vi "main.vi"() -> ()   [LabVIEW 2018]
uses:
  typedefs/measurement_settings.ctl
  typedefs/device_details.ctl
  typedefs/state_selector.ctl
  <instrlib>/Keithley 24XX/Public/Data/Read (Multiple Points).vi
  <instrlib>/Keithley 24XX/Keithley 24XX.lvlib
panel:
  out "timestamp":string
  out "experiment folder":path
  out "settings path":path
  out "Pixel data file":path
  in  "Tab Control":enum32{"Settings", "Measurement", "Advanced"}(tab)
  in  "Device details":T1={"Device label"="", "Pixel"=enum."1", "Area (cm^2)"=0.0}
  out "Username":string
  out "Experiment Name":string
  in  "Measurement settings":T2={"Minimum LED current (A)"=0.001, "Maximum LED Current (A)"=0.7, "Number of LED currents in sweep"=20, "LED current sweep mode"=1, "LED current sweep direction"=0, "LED settling delay (ms)"=500, "Solar cell measurement mode"=0, "Minimum JV voltage (V)"=-1.2, "Maximum JV voltage (V)"=0.1, "JV voltage step (V)"=0.02, "JV sweep direction"=0, "Dual JV sweep"=1, "Current range"=0, "Voltage range"=2, "Integration time (NPLC)"=1, "Auto settling delay"=1, "Settling delay (ms)"=3.0, "Enable display"=0} {"Voltage range" items=["Auto", "200 mV", "2.1 V", "21 V", "210 V"]; "Enable display" items=["False", "True"]; "Auto settling delay" items=["False", "True"]; "Settling delay (ms)" min=0.2 max=999999.9; "Integration time (NPLC)" items=["0.01", "0.1", "1", "10"]; "Current range" items=["Auto", "1 uA", "10 uA", "100 uA", "1 mA", "10 mA", "100 mA", "1 A"]; "Dual JV sweep" items=["False", "True"]; "JV sweep direction" items=["Ascending", "Descending"]; "JV voltage step (V)" min=0.0001 max=5.0 step=0.0001; "Solar cell measurement mode" items=["J-V", "Voc", "Jsc"]; "LED current sweep direction" items=["Ascending", "Descending"]; "LED current sweep mode" items=["Linear", "Logarithmic"]; "Maximum LED Current (A)" min=0.0 max=0.7 step=0.001 format="%#.3f"; "Minimum LED current (A)" min=0.0 max=0.7 step=0.001 format="%#.3f"}
  in  "Scan":bool
  in  "Initialise instruments":bool
  in  "Stop scan":bool
  out "TTi Power Supply":bool
  out "Pixel Selector":bool
  in  "Exit":bool
  out "Kiethley 2400":bool
  in  "LED current (A)":dbl=0.1 min=0.0 max=0.5
  in  "Pixel":u16=1
  out "Light on":bool
  in  "Toggle white light":bool
  in  "Keithley Address":refnum<visa-resource-name>="GPIB0::8::INSTR"
  in  "TTi QL564P":refnum<visa-resource-name>="COM6"
  in  "Set switch":bool
  in  "Tab Control 2":enum32{"Page 1"}(tab)
  out "Graph":cluster{"Voltage":dbl[], dbl[]}[](graph)
  # "Intensity Dependence"
  # "1."
  # "4."
  # "5."
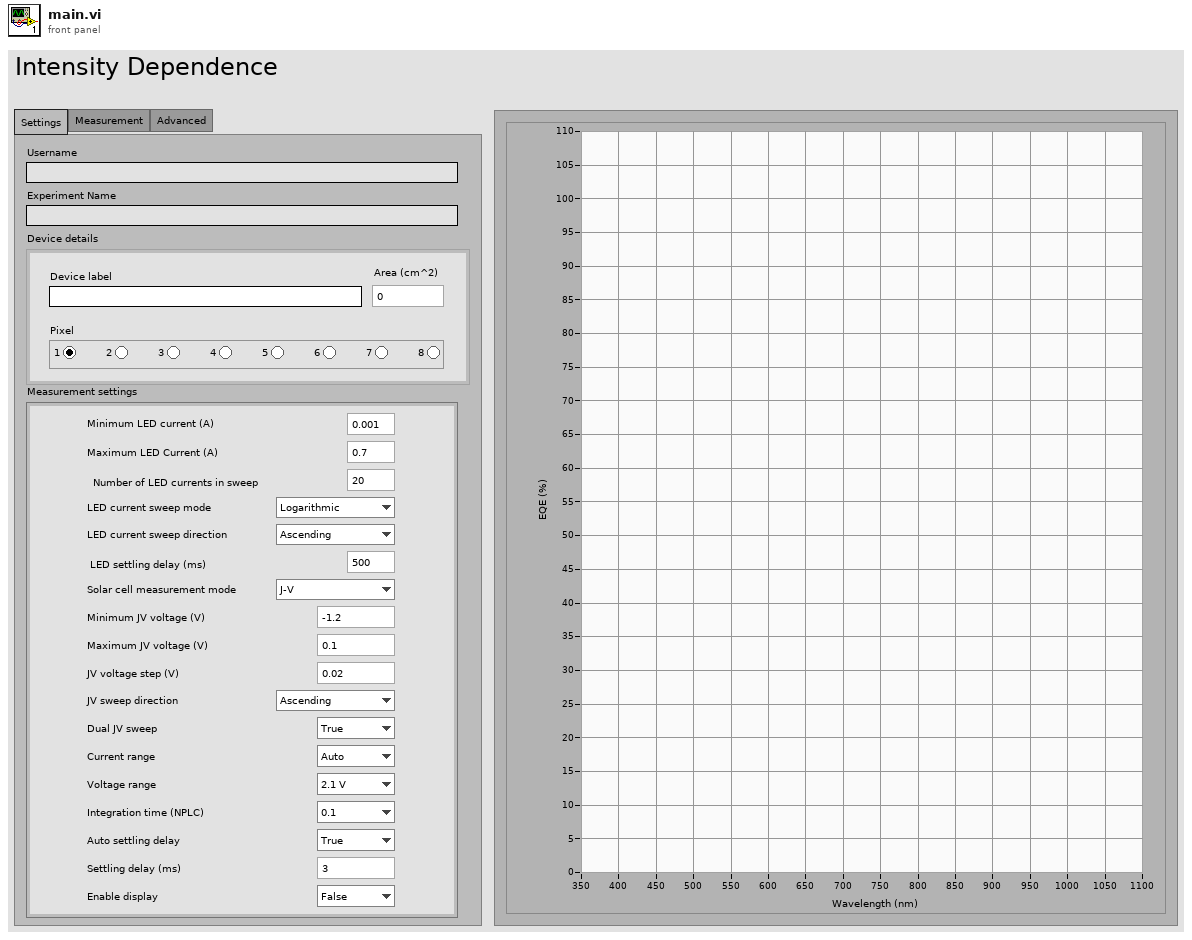
[diagram p1: front panel]
types:
  T1 = typedef "device_details.ctl" = cluster{"Device label":string, "Pixel":enum32{"No Selection", "1", "2", "3", "4", "5", "6", "7", "8"}, "Area (cm^2)":dbl}
  T2 = typedef "measurement_settings.ctl" = cluster{"Minimum LED current (A)":dbl, "Maximum LED Current (A)":dbl, "Number of LED currents in sweep":u32, "LED current sweep mode":u16, "LED current sweep direction":u16, "LED settling delay (ms)":u32, "Solar cell measurement mode":u16, "Minimum JV voltage (V)":dbl, "Maximum JV voltage (V)":dbl, "JV voltage step (V)":dbl, "JV sweep direction":u16, "Dual JV sweep":u16, "Current range":u16, "Voltage range":u16, "Integration time (NPLC)":u16, "Auto settling delay":u16, "Settling delay (ms)":dbl, "Enable display":u16}
  T3 = typedef "state_selector.ctl" = enum16{"Initialise software", "Idle", "Initialise instruments", "Scan", "Exit"}
  T4 = enum8{"Enabled", "Disabled", "Disabled and Grayed Out"}
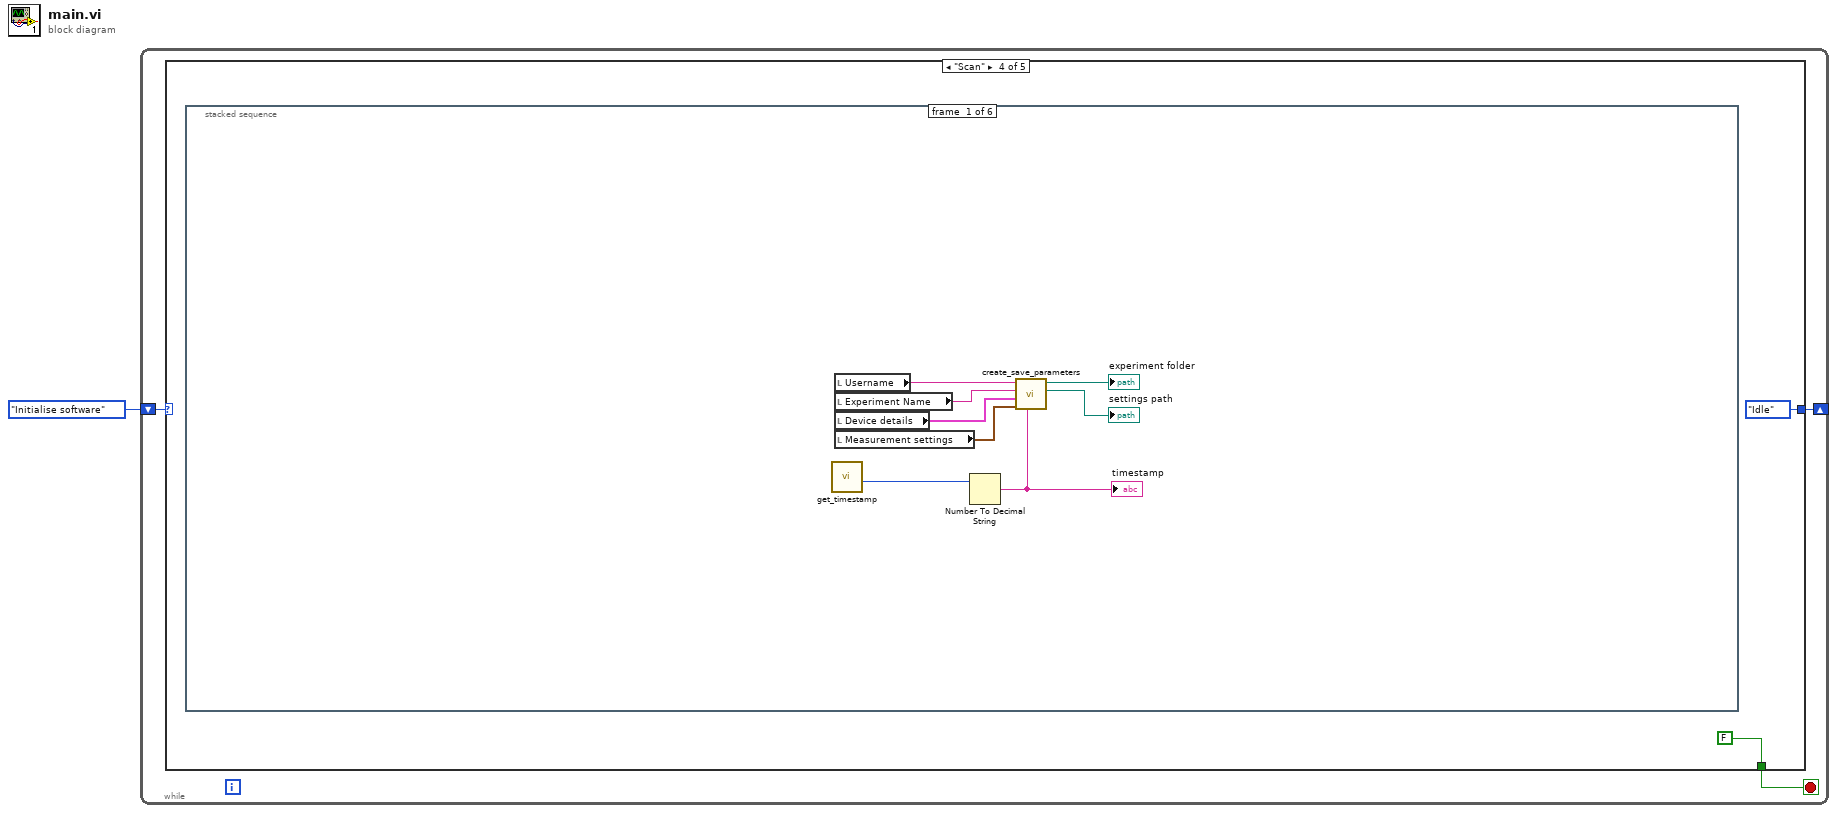
[diagram p0: block diagram]
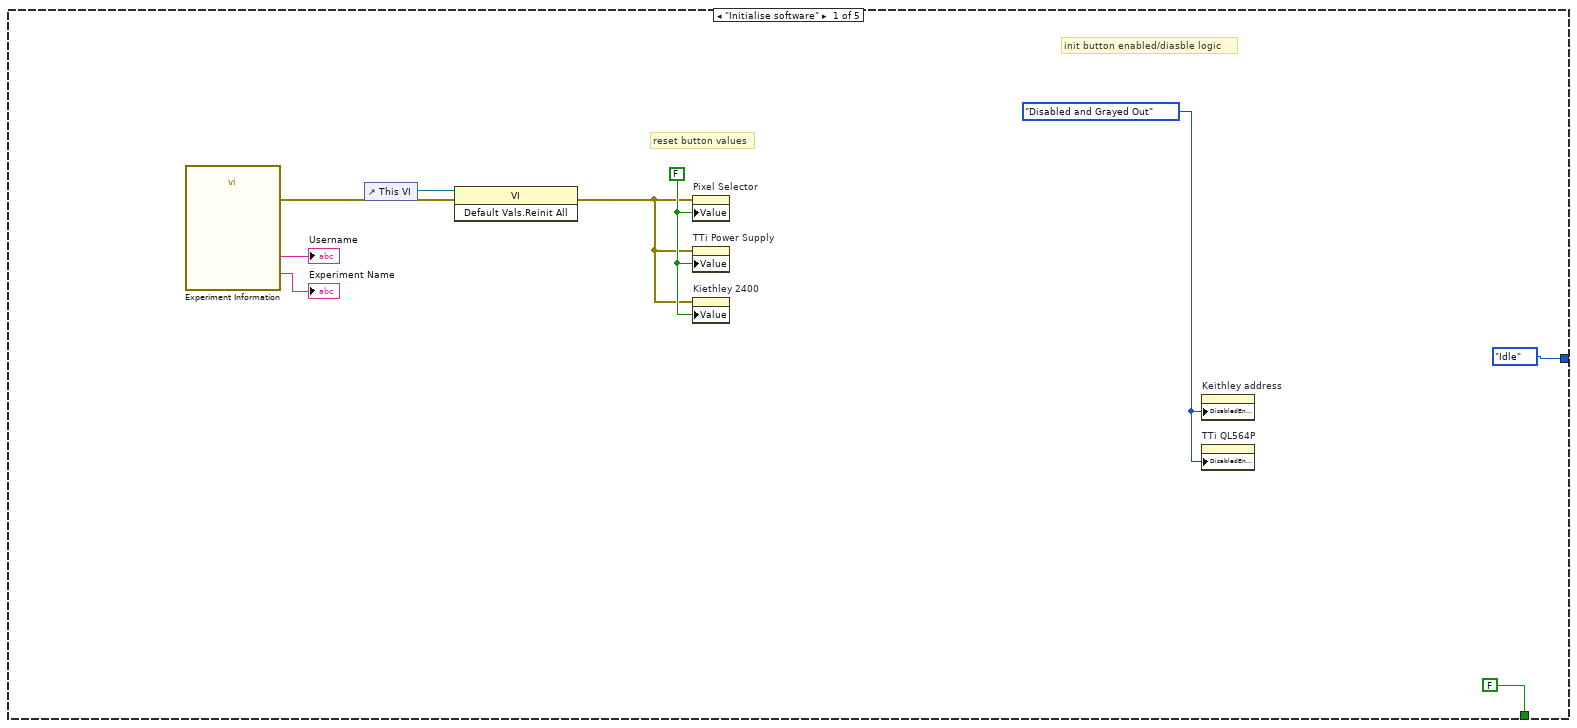
[diagram p2: hidden frame]
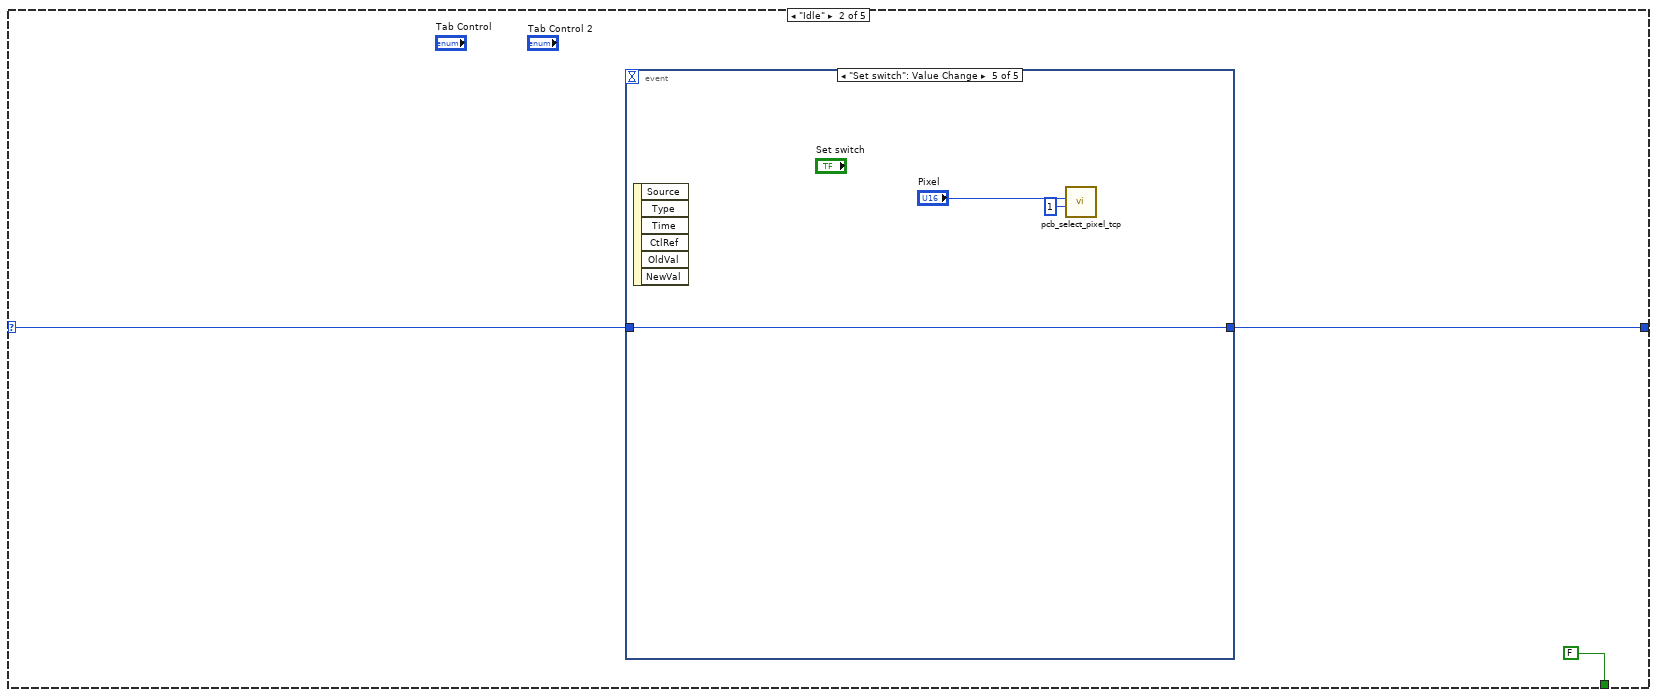
[diagram p3: hidden frame]
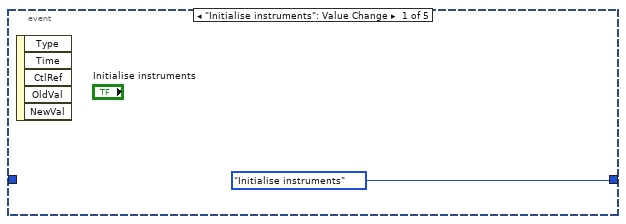
[diagram p4: hidden frame]
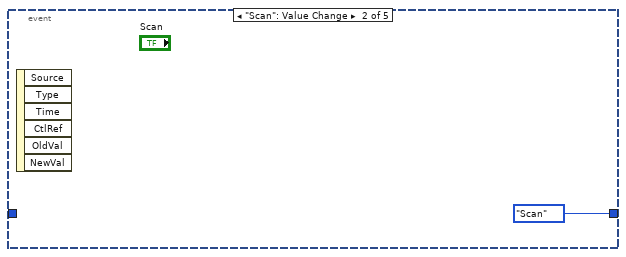
[diagram p5: hidden frame]
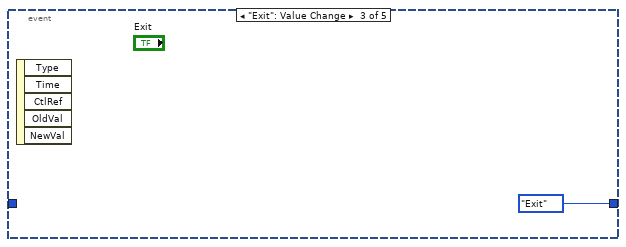
[diagram p6: hidden frame]
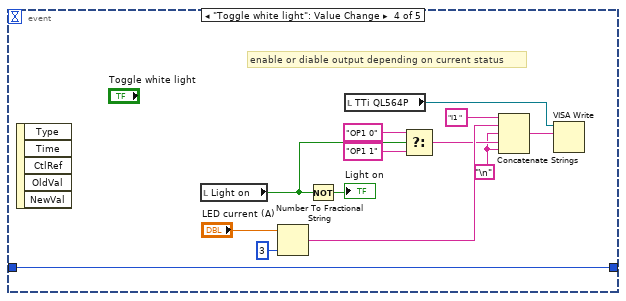
[diagram p7: hidden frame]
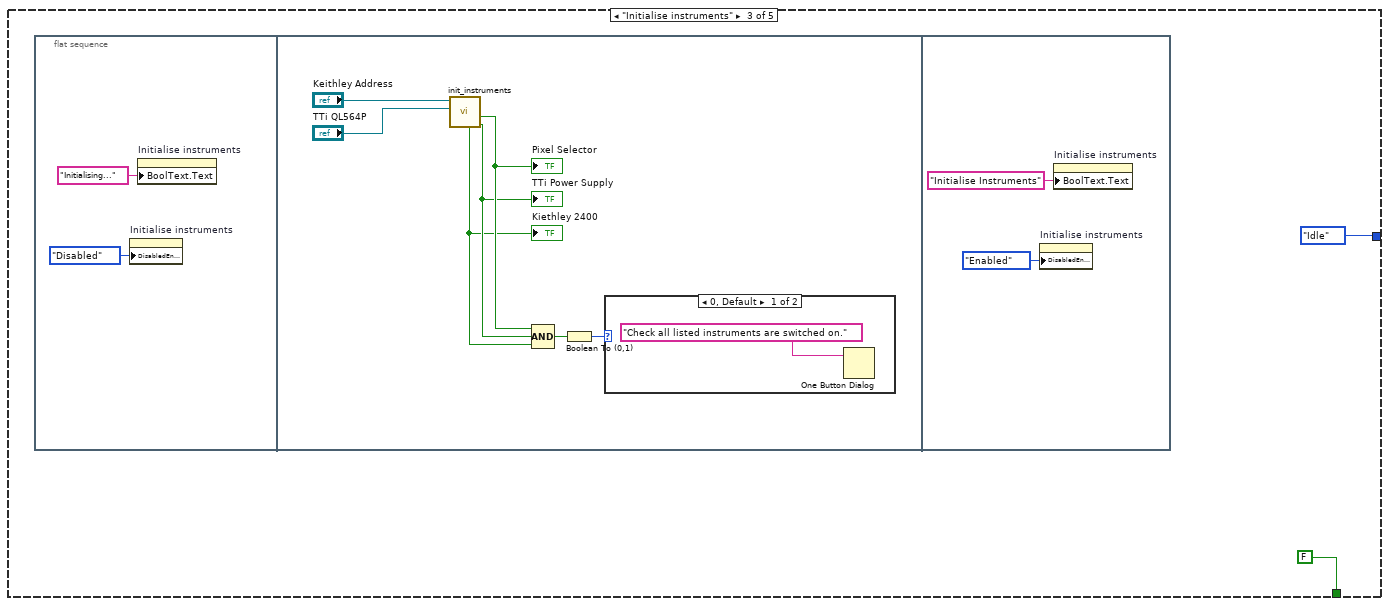
[diagram p8: hidden frame]
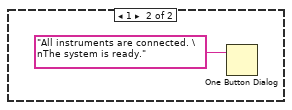
[diagram p9: hidden frame]
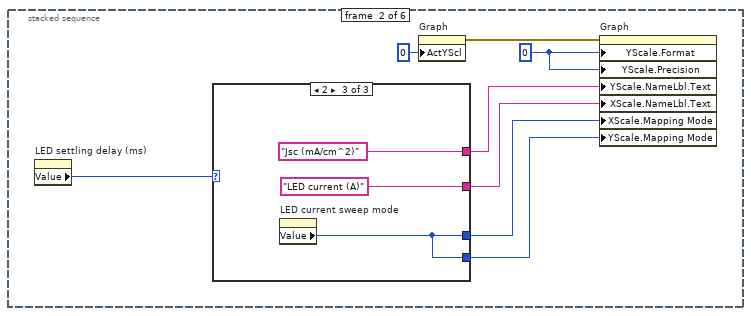
[diagram p10: hidden frame]
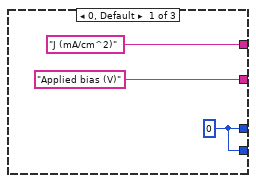
[diagram p11: hidden frame]
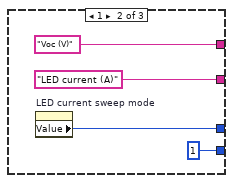
[diagram p12: hidden frame]
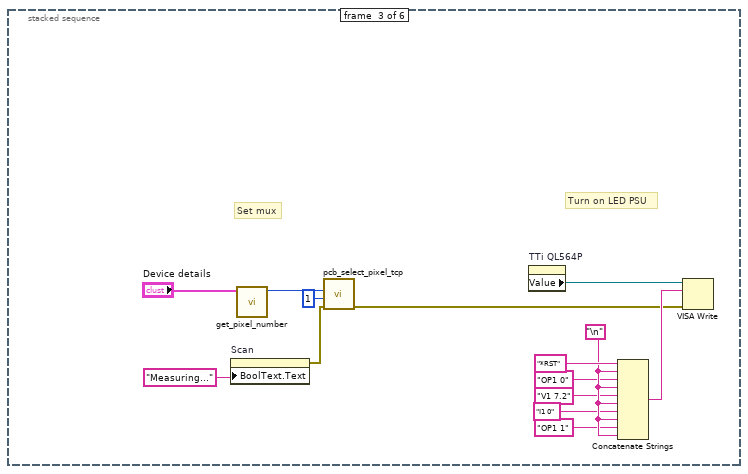
[diagram p13: hidden frame]
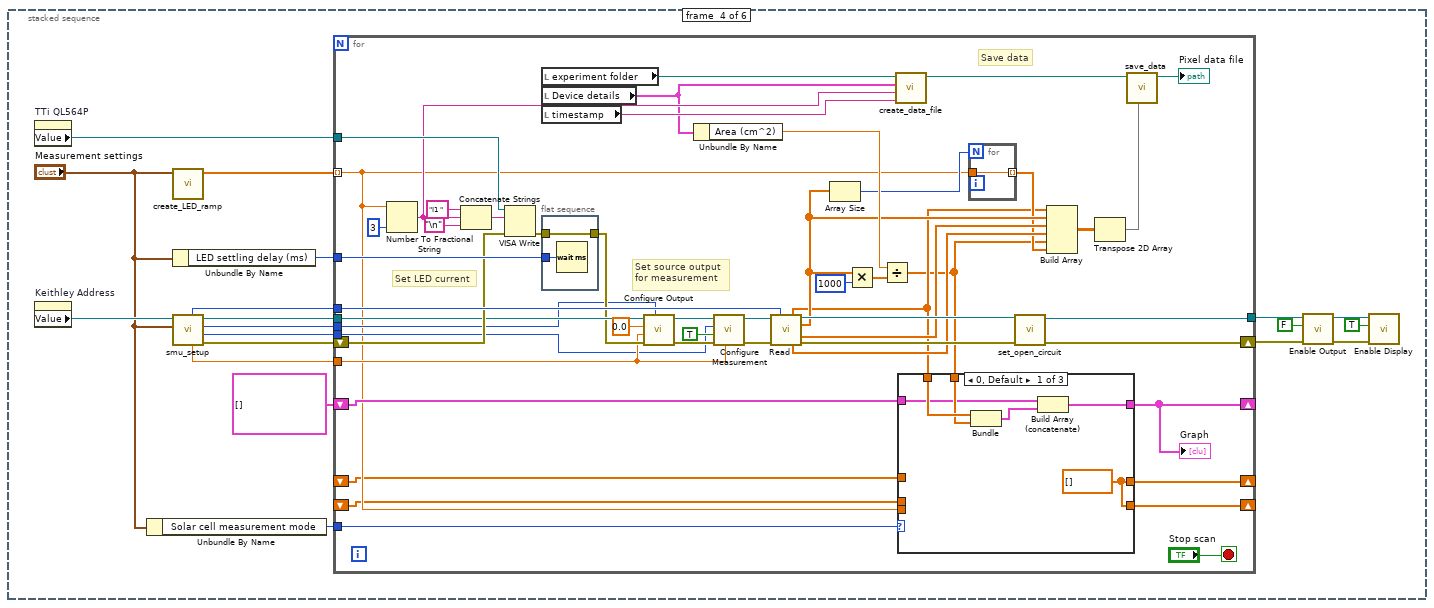
[diagram p14: hidden frame]
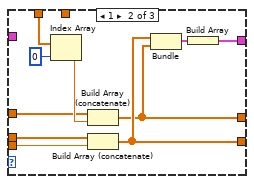
[diagram p15: hidden frame]
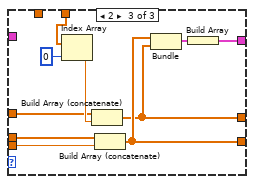
[diagram p16: hidden frame]
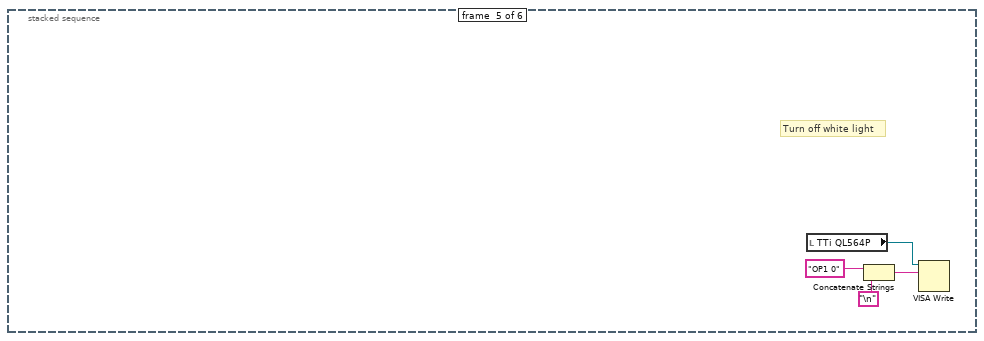
[diagram p17: hidden frame]
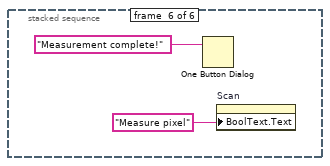
[diagram p18: hidden frame]
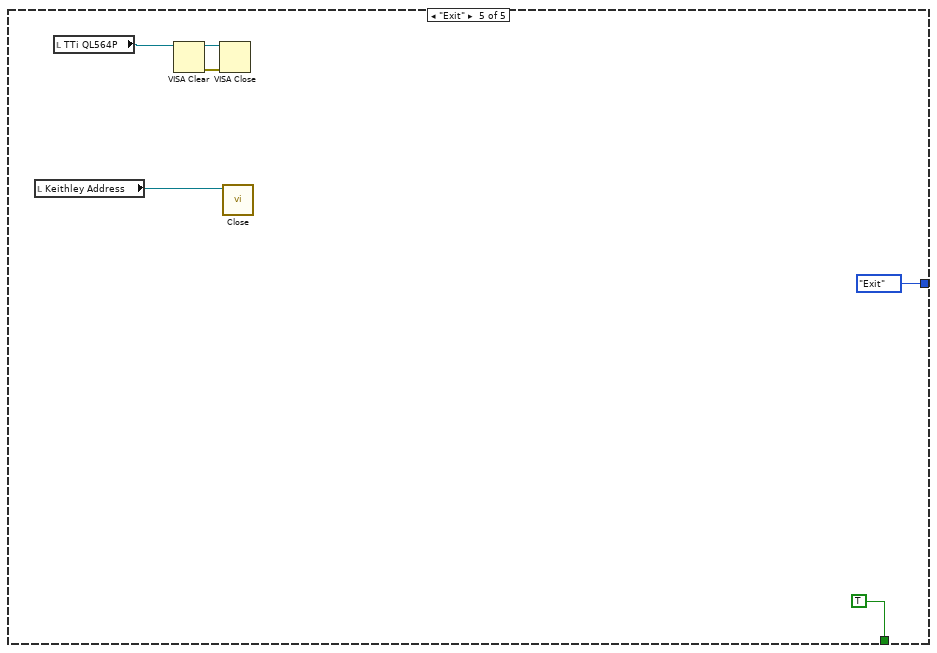
[diagram p19: hidden frame]
diagram:
  n1 = while {
    shift-right: [w3] -> _
    shift-left: state_selector."Initialise software" ("Enum") -> [w4]
    stop <- w2 stop-if-true
    n2 = case shown="\"Scan\"" w4 {
      selector: w4 -> [_ w15 _ _ _]
      tunnel: [state_selector."Idle" ("Enum") w16 state_selector."Idle" ("Enum") state_selector."Idle" ("Enum") state_selector."Exit" ("Enum")] -> w3
      tunnel: [FALSE FALSE FALSE FALSE TRUE] -> w2
      frame "Initialise software" {
        w8 = T4."Disabled and Grayed Out" ("Disabled")
        w9 = FALSE ("Scan")
        # "init button enabled/diasble logic"
        # "reset button values"
        n3 = call "Experiment Information"() -> ("Experiment Title"=→"Experiment Name":string, "Username"=→"Username":string, "error out"=w6:errorcluster)  [unwired: 16 in, 1 out]
        n4 = control-ref of="This VI"() -> (w7:refnum<vi>)
        n5 = invoke class="VI" method="Default Vals.Reinit All"(reference=w7, error in=w6) -> (error out=w5:errorcluster)  [unwired: 1 in, 2 out]
        n6 = property on="Pixel Selector" class="Bool (strict)"(error in=w5, "Value"=w9) -> ()  [unwired: 1 in, 2 out]
        n7 = property on="TTi Power Supply" class="Bool (strict)"(error in=w5, "Value"=w9) -> ()  [unwired: 1 in, 2 out]
        n8 = property on="Kiethley 2400" class="Bool (strict)"(error in=w5, "Value"=w9) -> ()  [unwired: 1 in, 2 out]
        n9 = property on="Keithley address" class="VISAName"("DisabledEnum"=w8) -> ()  [unwired: 2 in, 2 out]
        n10 = property on="TTi QL564P" class="VISAName"("DisabledEnum"=w8) -> ()  [unwired: 2 in, 2 out]
      }
      frame "Idle" {
        n11 = event shown="[4] \"Set switch\": Value Change" {
          selector: _ -> [_ _ _ _ _]
          dyn-events: _ -> [_ _ _ _ _]
          timeout: _ -> [_ _ _ _ _]
          tunnel: w15 -> [_ _ _ w32 w35]
          tunnel: [state_selector."Initialise instruments" ("Enum") state_selector."Scan" ("Enum") state_selector."Exit" ("Enum") w32 w35] -> w16
          event "Initialise instruments": Value Change {
            n12 = event-data() -> ()  [unwired: 1 in, 5 out]
          }
          event "Scan": Value Change {
            n13 = event-data() -> ()  [unwired: 1 in, 6 out]
          }
          event "Exit": Value Change {
            n14 = event-data() -> ()  [unwired: 1 in, 5 out]
          }
          event "Toggle white light": Value Change {
            w20 = "\n"
            # "enable or diable output depending on current status"
            n15 = event-data() -> ()  [unwired: 1 in, 5 out]
            n16 = local read "Light on"() -> (w27:bool)
            n17 = Number To Fractional String(number="LED current (A)", precision (6)=i16 3) -> (F-format string=w23:string)  [unwired: 2 in]
            n18 = Not(x=w27) -> (.not. x?=→"Light on":bool)
            n19 = local read "TTi QL564P"() -> (w26:refnum<visa-resource-name>)
            n20 = Select(t="OP1 0" ("Channel Name"), s=w27, f="OP1 1" ("Channel Name")) -> (s? t:f=w21:string)
            n21 = Concatenate Strings("I1 " ("Channel Name"), w23, w20, w21, w20) -> (w31:string)
            n22 = VISA Write(VISA resource name=w26, write buffer=w31) -> ()  [unwired: 1 in, 3 out]
          }
          event "Set switch": Value Change {
            n23 = event-data() -> ()  [unwired: 1 in, 6 out]
            n24 = call "pcb_select_pixel_tcp.vi"("Cell"=u32 1, "Pixel"="Pixel") -> ()  [unwired: 8 in, 2 out]
          }
        }
      }
      frame "Initialise instruments" {
        n25 = flat-sequence {
          frame #0 {
            n26 = property on="Initialise instruments" class="Bool"("DisabledEnum"=T4."Disabled" ("Disabled")) -> ()  [unwired: 2 in, 2 out]
            n27 = property on="Initialise instruments" class="Bool"("BoolText.Text"="Initialising..." ("Boolean Text.Text")) -> ()  [unwired: 2 in, 2 out]
          }
          frame #1 {
            n28 = call "init_instruments.vi"("LED PSU resource name"="TTi QL564P", "SMU resource name"="Keithley Address") -> ("LED power supply"=w43:bool, "Pixel Selector"=w44:bool, "SMU"=w42:bool)  [unwired: 7 in]
            "Kiethley 2400" <- w42
            "Pixel Selector" <- w44
            "TTi Power Supply" <- w43
            n29 = Compound Arithmetic op=AND(w44, w43, w42) -> (w46:bool)
            n30 = Boolean To (0,1)(Boolean=w46) -> (0, 1=w45:i16)
            n31 = case shown="0, Default" w45 {
              frame 0, Default {
                n32 = One Button Dialog(message="Check all listed instruments are switched on.") -> ()  [unwired: 1 in, 1 out]
              }
              frame 1 {
                n33 = One Button Dialog(message="All instruments are connected. \nThe system is ready.") -> ()  [unwired: 1 in, 1 out]
              }
            }
          }
          frame #2 {
            n34 = property on="Initialise instruments" class="Bool"("DisabledEnum"=T4."Enabled" ("Disabled")) -> ()  [unwired: 2 in, 2 out]
            n35 = property on="Initialise instruments" class="Bool"("BoolText.Text"="Initialise Instruments" ("Boolean Text.Text")) -> ()  [unwired: 2 in, 2 out]
          }
        }
      }
      frame "Scan" {
        n36 = stacked-sequence {
          frame #0 {
            n37 = call "get_timestamp.vi"() -> ("unix time (seconds since the epoch)"=w54:u32)  [unwired: 9 in, 2 out]
            n38 = local read "Username"() -> (w60:string)
            n39 = local read "Experiment Name"() -> (w59:string)
            n40 = local read "Device details"() -> (w58:T1)
            n41 = local read "Measurement settings"() -> (w57:T2)
            n42 = Number To Decimal String(number=w54) -> (decimal integer string=w53:string)  [unwired: 1 in]
            "timestamp" <- w53
            n43 = call "create_save_parameters.vi"("timestamp"=w53, "Measurement settings"=w57, "Device details"=w58, "Experiment Title"=w59, "Username"=w60) -> ("settings path"=→"settings path":path, "experiment folder"=→"experiment folder":path)  [unwired: 5 in]
          }
          frame #1 {
            w66 = u8 0 ("Y Scale.Display Format:Format")
            n44 = property on="LED settling delay (ms)" class="DigNum (strict)"() -> ("Value"=w65:u32)  [unwired: 2 in, 2 out]
            n45 = case shown="2" w65 {
              tunnel: ["J (mA/cm^2)" ("Y Scale.Name Label.Text") "Voc (V)" ("Y Scale.Name Label.Text") "Jsc (mA/cm^2)" ("Y Scale.Name Label.Text")] -> w64
              tunnel: ["Applied bias (V)" ("Y Scale.Name Label.Text") "LED current (A)" ("Y Scale.Name Label.Text") "LED current (A)" ("Y Scale.Name Label.Text")] -> w63
              tunnel: [w69 w73 w76] -> w62
              tunnel: [w69 1 w76] -> w61
              frame 0, Default {
                w69 = u16 0 ("Value")
              }
              frame 1 {
                n46 = property on="LED current sweep mode" class="Ring (strict)"() -> ("Value"=w73:u16)  [unwired: 2 in, 2 out]
              }
              frame 2 {
                n47 = property on="LED current sweep mode" class="Ring (strict)"() -> ("Value"=w76:u16)  [unwired: 2 in, 2 out]
              }
            }
            n48 = property on="Graph" class="XYGraph (strict)"("ActYScl"=0 ("Active Y Scale")) -> (error out=w68:errorcluster)  [unwired: 2 in, 1 out]
            n49 = property on="Graph" class="XYGraph (strict)"(error in=w68, "YScale.Format"=w66, "YScale.Precision"=w66, "YScale.NameLbl.Text"=w64, "XScale.NameLbl.Text"=w63, "XScale.Mapping Mode"=w62, "YScale.Mapping Mode"=w61) -> ()  [unwired: 1 in, 2 out]
          }
          frame #2 {
            w85 = "\n"
            # "Turn on LED PSU"
            # "Set mux"
            n50 = property on="Scan" class="Bool"("BoolText.Text"="Measuring..." ("Boolean Text.Text")) -> (error out=w90:errorcluster)  [unwired: 2 in, 1 out]
            n51 = call "get_pixel_number.vi"("Device details"="Device details") -> ("Pixel"=w89:i32)  [unwired: 9 in, 1 out]
            n52 = call "pcb_select_pixel_tcp.vi"("error in (no error)"=w90, "Cell"=u32 1, "Pixel"=w89) -> ("error out"=w80:errorcluster)  [unwired: 7 in, 1 out]
            n53 = property on="TTi QL564P" class="VISAName"() -> ("Value"=w79:refnum<visa-resource-name>)  [unwired: 2 in, 2 out]
            n54 = Concatenate Strings("*RST" ("string"), w85, "OP1 0" ("string"), w85, "V1 7.2" ("string"), w85, "I1 0" ("string"), w85, "OP1 1" ("string"), w85) -> (w87:string)
            n55 = VISA Write(VISA resource name=w79, write buffer=w87, error in (no error)=w80) -> ()  [unwired: 3 out]
          }
          frame #3 {
            n56 = property on="TTi QL564P" class="VISAName"() -> ("Value"=w96:refnum<visa-resource-name>)  [unwired: 2 in, 2 out]
            n57 = property on="Keithley Address" class="VISAName"() -> ("Value"=w110:refnum<visa-resource-name>)  [unwired: 2 in, 2 out]
            n58 = Unbundle By Name("Measurement settings") -> ("Solar cell measurement mode"=w94:u16)
            n59 = call "create_LED_ramp.vi"("Measurement settings"="Measurement settings") -> ("Ramp Pattern"=w111:dbl[])  [unwired: 10 in]
            n60 = Unbundle By Name("Measurement settings") -> ("LED settling delay (ms)"=w108:u32)
            n61 = call "smu_setup.vi"("Measurement settings"="Measurement settings", "VISA Refnum in"=w110) -> ("error out"=w107:errorcluster, "Measure Mode"=w102:u16, "Source Mode"=w103:u16, "VISA resource name out"=w106:refnum<visa-resource-name>, "Range"=w104:dbl, "samples"=w105:i32)  [unwired: 4 in]
            n62 = for {
              tunnel: w111 -> [w116] mode=indexing
              shift-right: [w139] -> w100
              shift-left: w107 -> [w150]
              tunnel: w108 -> [w156]
              tunnel: w106 -> [w149]
              tunnel: w105 -> [w155]
              tunnel: w104 -> [w147]
              tunnel: w103 -> [w146]
              tunnel: w102 -> [w145]
              tunnel: [w140] -> w101
              tunnel: w96 -> [w138]
              shift-right: [w118] -> _
              shift-left: cluster{"Voltage":sgl[], dbl[]}[] [] -> [w119]
              tunnel: w94 -> [w117]
              shift-right: [w115] -> _
              shift-left: _ -> [w114]
              shift-right: [w113] -> _
              shift-left: _ -> [w112]
              stop <- "Stop scan" stop-if-true
              # "Save data"
              # "Set LED current"
              # "Set source output\nfor measurement"
              n63 = Number To Fractional String(number=w116, precision (6)=i16 3) -> (F-format string=w133:string)  [unwired: 2 in]
              n64 = Concatenate Strings("I1 " ("string"), w133, "\n") -> (w161:string)
              n65 = VISA Write(VISA resource name=w138, write buffer=w161, error in (no error)=w150) -> (error out=w157:errorcluster)  [unwired: 2 out]
              n66 = local read "experiment folder"() -> (w135:path)
              n67 = local read "Device details"() -> (w132:T1)
              n68 = local read "timestamp"() -> (w134:string)
              n69 = flat-sequence {
                tunnel: w157 -> [w191]
                tunnel: [w191] -> w148
                tunnel: w156 -> [w190]
                frame #0 {
                  n70 = Wait (ms)(milliseconds to wait=w190) -> ()  [unwired: 1 out]
                }
              }
              n71 = call <instrlib>:"Configure Output.vi"("Source Mode  (0: Voltage)"=w146, "error in (no error)"=w148, "Compliance  Level (0.1)"=w147, "Output Level (0)"=0.0, "VISA resource name"=w149) -> ("error out"=w153:errorcluster, "VISA resource name out"=w154:refnum<visa-resource-name>)  [unwired: 1 in, 4 out]
              n72 = Unbundle By Name(w132) -> ("Area (cm^2)"=w129:dbl)
              n73 = call <instrlib>:"Configure Measurement.vi"("Manual Range (1.0)"=w147, "error in (no error)"=w153, "Enable Auto Range (T:Enable)"=TRUE, "Function (0: Volts)"=w145, "VISA resource name"=w154) -> ("error out"=w143:errorcluster, "VISA resource name out"=w144:refnum<visa-resource-name>)  [unwired: 5 out]
              n74 = call-poly <instrlib>:"Read.vi"("VISA resource name"=w144, "Sample Count (1)"=w155, "error in (no error)"=w143) -> ("Voltage"=w121:sgl[], "VISA resource name out"=w142:refnum<visa-resource-name>, "Current"=w123:sgl[], "Timestamp"=w128:sgl[], "Status"=w127:sgl[], "error out"=w141:errorcluster)  [unwired: 2 in, 5 out]
              n75 = Array Size(array=w123) -> (size(s)=w124:i32)
              n76 = Multiply(x=w123, y=1000) -> (x*y=w130:sgl[])
              n77 = Divide(x=w129, y=w130) -> (x/y=w120:dbl[])
              n78 = call "create_data_file.vi"("timestamp"=w134, "LED current (A)"=w133, "Device details"=w132, "experiment folder"=w135) -> ("Filepath out"=w137:path)  [unwired: 7 in]
              n79 = case shown="0, Default" w117 {
                tunnel: w121 -> [w168 w176 _]
                tunnel: w120 -> [w167 _ w179]
                tunnel: w119 -> [w165 _ _]
                tunnel: [w164 w177 w187] -> w118
                tunnel: w116 -> [_ w174 w185]
                tunnel: [w163 w170 w181] -> w115
                tunnel: w114 -> [_ w173 w184]
                tunnel: [w163 w169 w180] -> w113
                tunnel: w112 -> [_ w171 w182]
                frame 0, Default {
                  w163 = dbl[] []
                  n80 = Bundle("Voltage"=w168, w167) -> (w166:cluster{"Voltage":sgl[], dbl[]})  [unwired: 1 in]
                  n81 = Build Array (concatenate)(w165, w166) -> (w164:cluster{"Voltage":dbl[], dbl[]}[])
                }
                frame 1 {
                  n82 = Index Array(array=w176, index=0) -> (element=w172:sgl)
                  n83 = Build Array (concatenate)(w171, w172) -> (w169:dbl[])
                  n84 = Build Array (concatenate)(w173, w174) -> (w170:dbl[])
                  n85 = Bundle(w170, w169) -> (w178:cluster{dbl[], dbl[]})  [unwired: 1 in]
                  n86 = Build Array(w178) -> (w177:cluster{dbl[], dbl[]}[])
                }
                frame 2 {
                  n87 = Index Array(array=w179, index=0) -> (element=w183:dbl)
                  n88 = Build Array (concatenate)(w182, w183) -> (w180:dbl[])
                  n89 = Build Array (concatenate)(w184, w185) -> (w181:dbl[])
                  n90 = Bundle(w181, w180) -> (w188:cluster{dbl[], dbl[]})  [unwired: 1 in]
                  n91 = Build Array(w188) -> (w187:cluster{dbl[], dbl[]}[])
                }
              }
              "Graph" <- w118
              n92 = for {
                N: w124 -> [_]
                tunnel: [w189] -> w122 mode=indexing
                tunnel: w116 -> [w189]
              }
              n93 = call "set_open_circuit.vi"("error in (no error)"=w141, "VISA Refnum in"=w142) -> ("error out"=w139:errorcluster, "VISA Refnum out"=w140:refnum<visa-resource-name>)  [unwired: 8 in]
              n94 = Build Array(w121, w123, w128, w127, w120, w122) -> (w126:dbl[][])
              n95 = Transpose 2D Array(2D array=w126) -> (transposed array=w125:dbl[][])
              n96 = call "save_data.vi"("data"=w125, "Filepath in"=w137) -> ("Filepath out"=→"Pixel data file":path)  [unwired: 9 in]
            }
            n97 = call <instrlib>:"Enable Output.vi"("error in (no error)"=w100, "Enable Output (T: Enable)"=FALSE, "VISA resource name"=w101) -> ("error out"=w98:errorcluster, "VISA resource name out"=w99:refnum<visa-resource-name>)  [unwired: 7 in]
            n98 = call <instrlib>:"Enable Display.vi"("error in (no error)"=w98, "Enable Display (T: Enable)"=TRUE, "VISA resource name"=w99) -> ()  [unwired: 9 out]
          }
          frame #4 {
            # "Turn off white light"
            n99 = local read "TTi QL564P"() -> (w192:refnum<visa-resource-name>)
            n100 = Concatenate Strings("OP1 0" ("Channel Name"), "\n") -> (w194:string)
            n101 = VISA Write(VISA resource name=w192, write buffer=w194) -> ()  [unwired: 1 in, 3 out]
          }
          frame #5 {
            n102 = One Button Dialog(message="Measurement complete!") -> ()  [unwired: 1 in, 1 out]
            n103 = property on="Scan" class="Bool"("BoolText.Text"="Measure pixel" ("Boolean Text.Text")) -> ()  [unwired: 2 in, 2 out]
          }
        }
      }
      frame "Exit" {
        n104 = local read "Keithley Address"() -> (w198:refnum<visa-resource-name>)
        n105 = local read "TTi QL564P"() -> (w199:refnum<visa-resource-name>)
        n106 = VISA Clear(VISA resource name=w199) -> (VISA resource name out=w201:refnum<visa-resource-name>, error out=w200:errorcluster)  [unwired: 1 in]
        n107 = VISA Close(VISA resource name=w201, error in (no error)=w200) -> ()  [unwired: 1 out]
        n108 = call <instrlib>:"Close.vi"("VISA resource name"=w198) -> ()  [unwired: 10 in, 1 out]
      }
    }
  }
